vi "Replace Data.vi"(6 "Index in":i32, 8 "error in (no error)":errorcluster, 9 "Value":string, 10 "Data":T1=enum."type", 11 "Composite Object in":refnum<class "CConfig Object.lvclass">) -> (0 "error out":errorcluster, 3 "Composite Object out":refnum<class "CConfig Object.lvclass">)   [LabVIEW 2013, in "CConfig Object.lvclass"]
doc: "Copyright 2018, Carya Automatisering, Wiebe Walstra."
uses:
  CConfig Object.lvclass
  Data.ctl
  CConfig Object.lvclass/CConfig Object.ctl
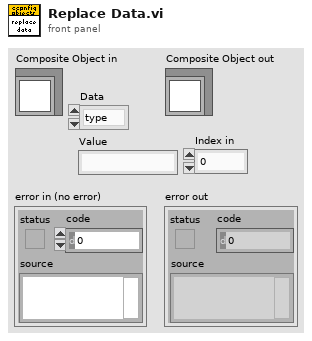
[diagram p1: front panel]
types:
  T1 = typedef "CConfig Object.lvclass/Data.ctl" = enum16{"pre", "name", "middle", "value", "post", "newline", "persistant", "tagged", "type"}
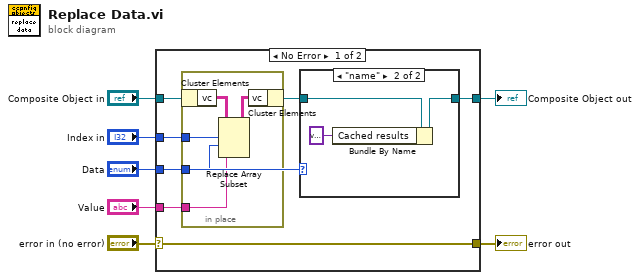
[diagram p0: block diagram]
diagram:
  n1 = case shown="No Error" "error in (no error)" {
    selector: "error in (no error)" -> [w14 w25]
    tunnel: [w14 w25] -> w6
    tunnel: [w8 w24] -> w4
    tunnel: "Composite Object in" -> [w13 w24]
    tunnel: "Index in" -> [w12 _]
    tunnel: "Value" -> [w11 _]
    tunnel: "Data" -> [w10 _]
    frame No Error {
      n2 = in-place {
        in-place-border: w12 -> [w21]
        in-place-border: w11 -> [w20]
        in-place-border: w10 -> [w19]
        n3 = in-place-cluster #1(w13) -> ("vc"=w23:string[][])
        n4 = Replace Array Subset(array=w23, new element=w20, index (row)=w21, index (col)=w19) -> (w22:string[][])
        n5 = in-place-cluster #1("vc"=w22) -> (w9:refnum<class "CConfig Object.lvclass">)
      }
      n6 = case shown="\"name\"" w10 {
        tunnel: w9 -> [w15 w18]
        tunnel: [w15 w17] -> w8
        frame Default {
        }
        frame "name" {
          n7 = Bundle By Name(cluster=w18, "Cached results"=variant) -> (w17:refnum<class "CConfig Object.lvclass">)
        }
      }
    }
    frame Error {
    }
  }
  "error out" <- w6
  "Composite Object out" <- w4
